vi "Sync Reply.vi"(7 "Sender":refnum<class "Sender.lvclass">, 10 "Msg":refnum<class "Msg.lvclass">, 11 "Actor in":refnum<class "Actor.lvclass">) -> (3 "Actor out":refnum<class "Actor.lvclass">)   [LabVIEW 2020, in "jettl.lvlib" / "Actor.lvlib" / "Actor.lvclass"]
uses:
  Actor.lvclass
  Sender/Sender/Sender.lvclass
  Msg/Msg.lvclass
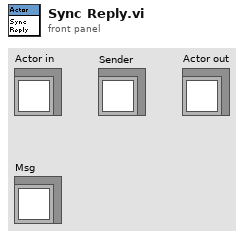
[diagram p1: front panel]
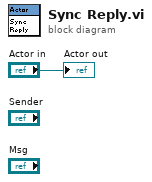
[diagram p0: block diagram]
diagram:
  "Actor out" <- "Actor in"
